vi "SVA 4MV6 P001 CCE rgb2gray.vi"(9 "B":u8, 10 "G":u8, 11 "R":u8) -> (3 "Escala grises":u8)   [LabVIEW 2020]
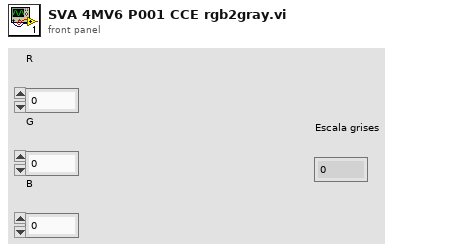
[diagram p1: front panel]
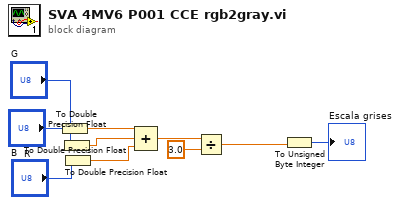
[diagram p0: block diagram]
diagram:
  n1 = To Double Precision Float(number="R") -> (double precision float=w8:dbl)
  n2 = To Double Precision Float(number="G") -> (double precision float=w7:dbl)
  n3 = To Double Precision Float(number="B") -> (double precision float=w6:dbl)
  n4 = Compound Arithmetic op=ADD(w8, w7, w6) -> (w10:dbl)
  n5 = Divide(x=w10, y=3.0) -> (x/y=w5:dbl)
  n6 = To Unsigned Byte Integer(number=w5) -> (unsigned 8bit integer=→"Escala grises":u8)
